vi "F Dwf Device Trigger Set.vi"(8 "error in (no error)":errorcluster, 9 "trigsrc":u8, 10 "idxPin":i32, 11 "hdwf":i32) -> (0 "error out":errorcluster, 3 "function return":i32)   [LabVIEW 2021, in "Olasdwf.lvlib"]
doc: "DWFAPI int FDwfDeviceTriggerInfo(HDWF hdwf, int *pfstrigsrc); DWFAPI int FDwfDeviceTriggerSet(HDWF hdwf, int idxPin, TRIGSRC trigsrc);"
uses:
  Olasdwf.lvlib
  Windows/System32/dwf.dll
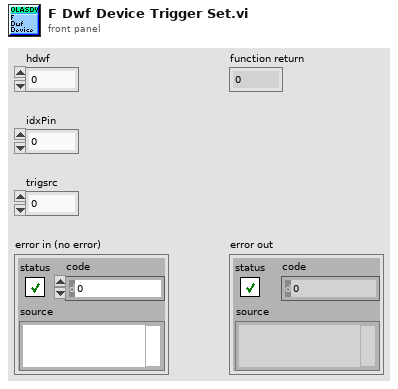
[diagram p1: front panel]
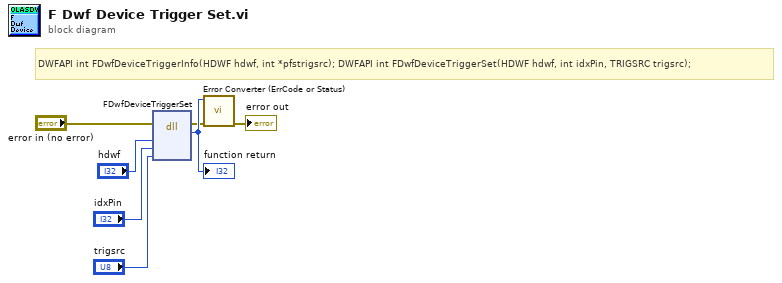
[diagram p0: block diagram]
diagram:
  # "DWFAPI int FDwfDeviceTriggerInfo(HDWF hdwf, int *pfstrigsrc); DWFAPI int FDwfDeviceTriggerSet(HDWF hdwf, int idxPin, TRIGSRC trigsrc);"
  n1 = dll-call lib="/Windows/System32/dwf.*" fn="FDwfDeviceTriggerSet"(error in="error in (no error)", "hdwf"="hdwf", "idxPin"="idxPin", "trigsrc"="trigsrc") -> (error out=w2:errorcluster, w7:i32)  [unwired: 5 in, 1 out]
  "function return" <- w7
  n2 = call "Error Converter (ErrCode or Status).vi"("error in (no error)"=w2, "error code"=w7) -> ("error out"=→"error out":errorcluster)  [unwired: 9 in]
